vi "Toggle Order.vi"(8 "error in (no error)":errorcluster, 9 "Column":i32, 10 "Display State In":T1, 11 "MCListbox Refnum in":refnum<vi>) -> (0 "error out":errorcluster, 2 "Display State Out":T1, 3 "MCListbox Refnum  out":refnum<vi>)   [LabVIEW 2012, in "ListBox_XControl.xctl"]
doc: "Toggles Display state order Between Ascending and Descending if the Column Header Row is re-clicked"
uses:
  ListBox_XControl.xctl
  ListBox_State.ctl
  Order Type Def.ctl
  Value Filters.ctl
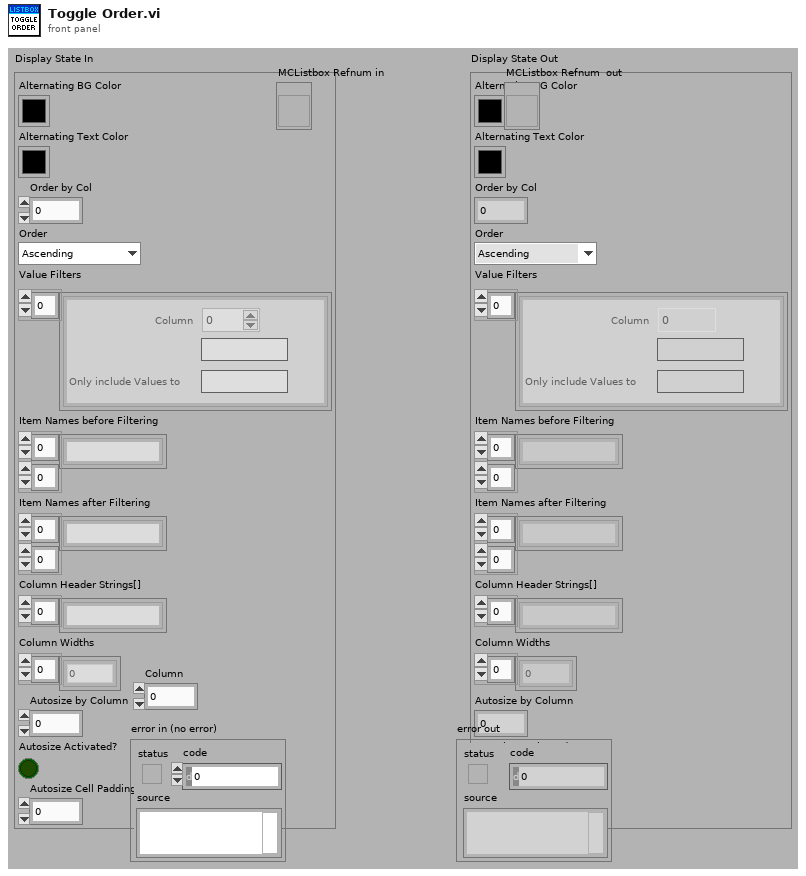
[diagram p1: front panel]
types:
  T1 = typedef "ListBox_XControl.xctl/ListBox_State.ctl" = cluster{"Alternating BG Color":u32, "Alternating Text Color":u32, "Order by Col":i32, "Order":T2, "Value Filters":T3, "Item Names before Filtering":string[][], "Item Names after Filtering":string[][], "Column Header Strings[]":string[], "Column Widths":u32[], "Autosize by Column":i32, "Autosize Activated?":bool, "Autosize Cell Padding":u32}
  T2 = typedef "ListBox_XControl.xctl/Order Type Def.ctl" = enum16{"Ascending", "Descending", "Off"}
  T3 = typedef "ListBox_XControl.xctl/Value Filters.ctl" = cluster{"Column":i32, "Only include Values From":string, "Only include Values to":string}[]
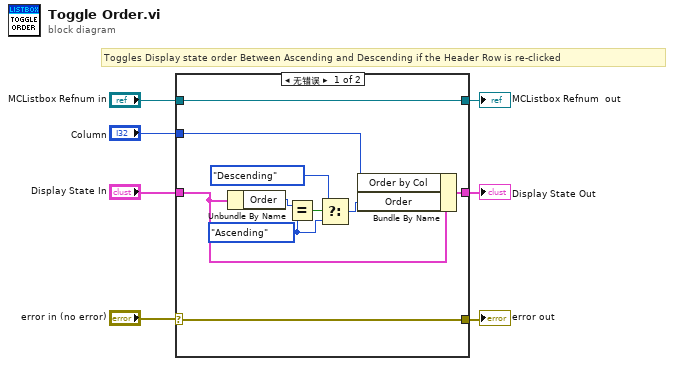
[diagram p0: block diagram]
diagram:
  # "Toggles Display state order Between Ascending and Descending if the Header Row is re-clicked"
  n1 = case shown="无错误" "error in (no error)" {
    selector: "error in (no error)" -> [w9 w20]
    tunnel: [w12 w19] -> w7
    tunnel: "Display State In" -> [w11 w19]
    tunnel: "Column" -> [w10 _]
    tunnel: [w9 w20] -> w3
    tunnel: [w8 w18] -> w2
    tunnel: "MCListbox Refnum in" -> [w8 w18]
    frame No Error {
      w15 = Order_Type_Def."Ascending" ("y")
      n2 = Unbundle By Name(w11) -> ("Order"=w13:T2)
      n3 = Equal?(x=w13, y=w15) -> (x = y?=w14:bool)
      n4 = Select(t=Order_Type_Def."Descending", s=w14, f=w15) -> (s? t:f=w17:T2)
      n5 = Bundle By Name(cluster=w11, "Order by Col"=w10, "Order"=w17) -> (w12:T1)
    }
    frame Error {
    }
  }
  "Display State Out" <- w7
  "error out" <- w3
  "MCListbox Refnum  out" <- w2
